vi "Decode.vi"(7 "Session Key":string, 8 "error in (no error)":errorcluster, 9 "Socket":string, 10 "Message In":string[](array[string]), 11 "object in":refnum<class "Message Class.lvclass">) -> (0 "error out":errorcluster, 1 "parent_header":T1={"msg_id"="", "username"="", "session"="", "date"=timestamp(0 s since 1904-01-01), "msg_type"="", "version"="5.0"}, 2 "Header":T1={"msg_id"="", "username"="", "session"="", "date"=timestamp(0 s since 1904-01-01), "msg_type"="", "version"="5.0"}, 3 "object out":refnum<class "Message Class.lvclass">, 4 "HMAC Signature":bool)   [LabVIEW 2018, in "ClientMessaging.lvlib" / "Message Class.lvclass"]
doc: "Decode a message and make a child class of the appropriate type"
uses:
  Message Class.lvclass
  protected/header_dict.ctl
  Message Class.lvclass/Message Class.ctl
  SHA256/SHA256.lvlib
  <vilib>/JDP Science/JSONtext/JSONtext.lvlib
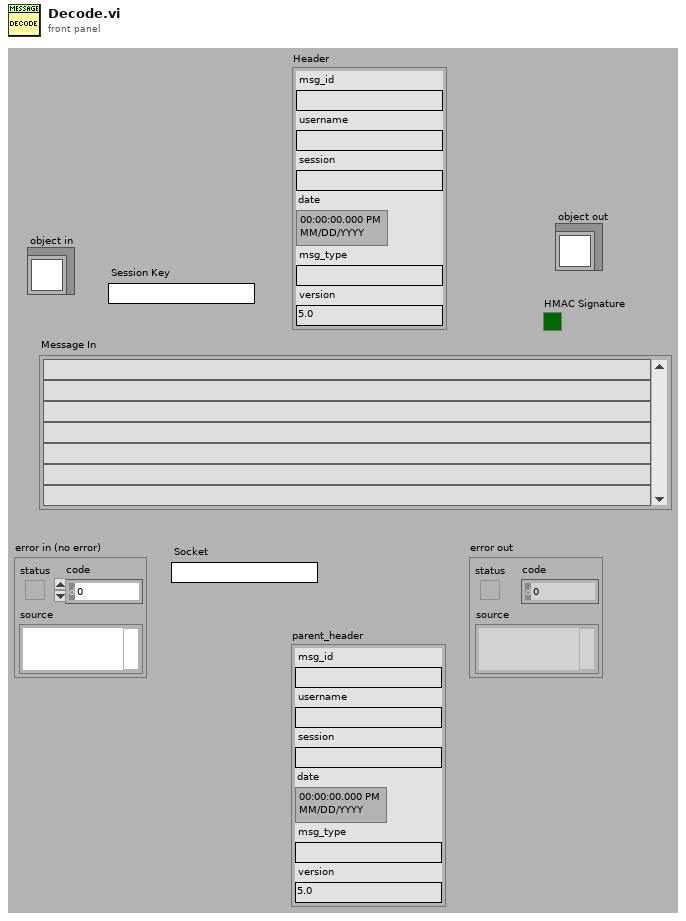
[diagram p1: front panel]
types:
  T1 = typedef "ClientMessaging.lvlib/Message Class.lvclass/header_dict.ctl" = cluster{"msg_id":string, "username":string, "session":string, "date":timestamp, "msg_type":string, "version":string}
  T2 = cluster{"[0]":string, "[1]":string, "[2]":string, "[3]":string}
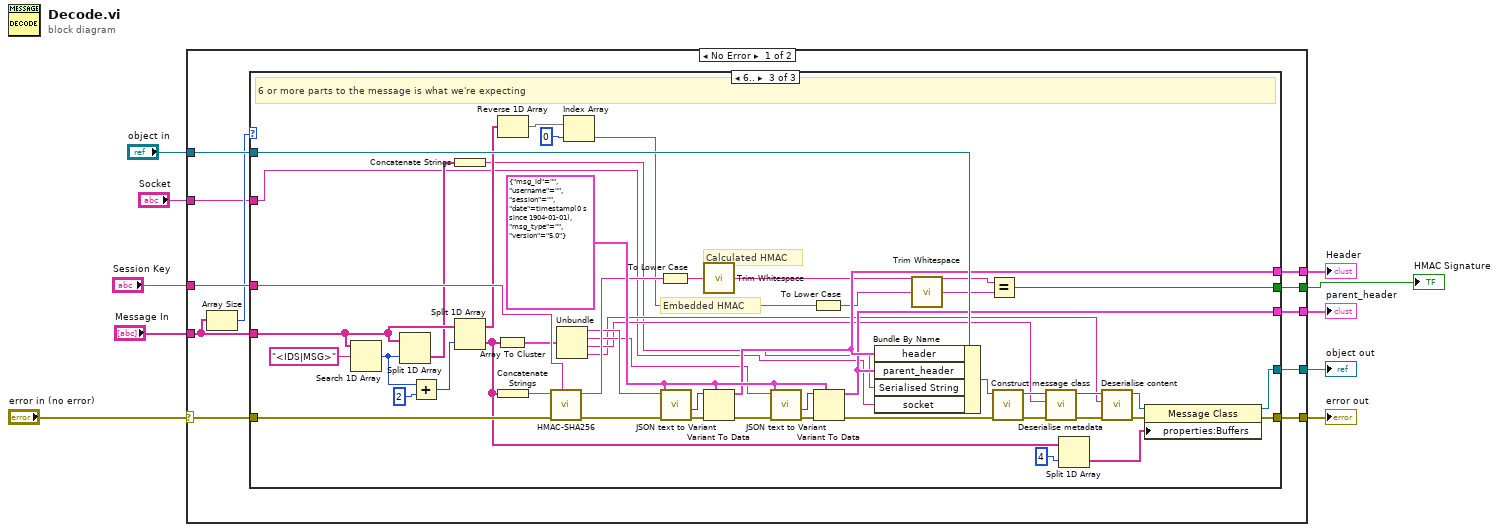
[diagram p0: block diagram]
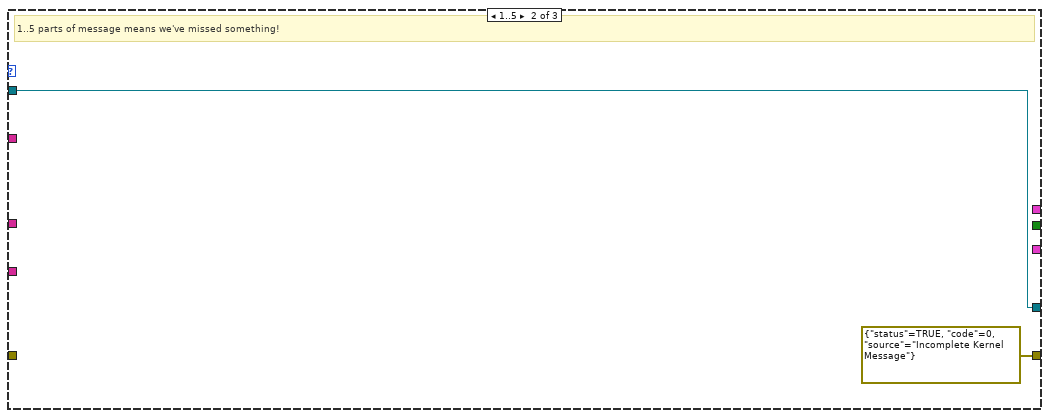
[diagram p3: hidden frame]
diagram:
  n1 = case shown="No Error" "error in (no error)" {
    selector: "error in (no error)" -> [w16 w76]
    tunnel: [w19 w76] -> w9
    tunnel: [w20 w75] -> w7
    tunnel: "object in" -> [w21 w75]
    tunnel: "Message In" -> [w13 _]
    tunnel: [w18 _] -> w5
    tunnel: [w17 _] -> w4
    tunnel: "Session Key" -> [w14 _]
    tunnel: [w15 _] -> w2
    tunnel: "Socket" -> [w11 _]
    frame No Error {
      n2 = Array Size(array=w13) -> (size(s)=w12:i32)
      n3 = case shown="6.." w12 {
        tunnel: w21 -> [w22 w25 w73]
        tunnel: [w22 w25 w59] -> w20
        tunnel: [w23 errorcluster {"status"=TRUE, "code"=0, "source"="Incomplete Kernel Message"} ("error out") w58] -> w19
        tunnel: [_ _ w57] -> w18
        tunnel: [_ _ w56] -> w17
        tunnel: w16 -> [w23 _ w55]
        tunnel: [_ _ w49] -> w15
        tunnel: w14 -> [_ _ w48]
        tunnel: w13 -> [_ _ w30]
        tunnel: w11 -> [_ _ w26]
        frame 0, Default {
          # "Ignore empty messages (probably just timeo out waiting for someone to talk to us)"
        }
        frame 1..5 {
          # "1..5 parts of message means we've missed something!"
        }
        frame 6.. {
          w66 = T1 {"msg_id"="", "username"="", "session"="", "date"=timestamp(0 s since 1904-01-01), "msg_type"="", "version"="5.0"} ("header")
          # "Calculated HMAC"
          # "Embedded HMAC"
          # "6 or more parts to the message is what we're expecting"
          n4 = Search 1D Array(1D array=w30, element="<IDS|MSG>" ("search string/char (-)")) -> (index of element=w29:i32)  [unwired: 1 in]
          n5 = Split 1D Array(array=w30, index=w29) -> (second subarray=w28:string[])  [unwired: 1 out]
          n6 = Add(x=w29, y=2) -> (x+y=w45:i32)
          n7 = Concatenate Strings(w28) -> (w27:string)
          n8 = Split 1D Array(array=w30, index=w45) -> (first subarray=w43:string[], second subarray=w33:string[])
          n9 = Array To Cluster(array=w33) -> (cluster=w39:T2)
          n10 = Reverse 1D Array(array=w43) -> (reversed array=w42:string[])
          n11 = Concatenate Strings(w33) -> (w47:string)
          n12 = call <vilib>:"HMAC-SHA256.vi"("Key"=w48, "error In"=w55, "String to Encode"=w47) -> ("error Out"=w46:errorcluster, "Hash String"=w54:string)  [unwired: 7 in]
          n13 = Unbundle(w39) -> ("[0]"=w38:string, "[1]"=w37:string, "[2]"=w36:string, "[3]"=w35:string)
          n14 = Index Array(array=w42, index=0) -> (element=w40:string)
          n15 = To Lower Case(string=w54) -> (all lower case string=w53:string)
          n16 = call <vilib>:"JSON text to Variant.vi"("error in (no error)"=w46, "Data Type"=w66, "JSON"=w38) -> ("error out"=w70:errorcluster, "Variant out"=w71:variant)  [unwired: 7 in]
          n17 = call <vilib>:"Trim Whitespace.vi"("string"=w53) -> ("trimmed string"=w51:string)  [unwired: 1 in]
          n18 = Variant To Data(error in=w70, type=w66, Variant=w71) -> (data=w57:T1, error out=w69:errorcluster)
          n19 = call <vilib>:"JSON text to Variant.vi"("error in (no error)"=w69, "Data Type"=w66, "JSON"=w37) -> ("error out"=w68:errorcluster, "Variant out"=w67:variant)  [unwired: 7 in]
          n20 = To Lower Case(string=w40) -> (all lower case string=w52:string)
          n21 = Variant To Data(error in=w68, type=w66, Variant=w67) -> (data=w56:T1, error out=w64:errorcluster)
          n22 = Bundle By Name(cluster=w73, "header"=w57, "parent_header"=w56, "Serialised String"=w27, "socket"=w26) -> (w72:refnum<class "Message Class.lvclass">)
          n23 = call <vilib>:"Trim Whitespace.vi"("string"=w52) -> ("trimmed string"=w50:string)  [unwired: 1 in]
          n24 = Equal?(x=w51, y=w50) -> (x = y?=w49:bool)
          n25 = call "Construct message class.vi"("error in (no error)"=w64, "object in"=w72) -> ("error out"=w63:errorcluster, "object out"=w65:refnum<class "Message Class.lvclass">)  [unwired: 8 in]
          n26 = call-dynamic "Deserialise metadata.vi"("error in (no error)"=w63, "JSON String to decode"=w36, "object in"=w65) -> ("error out"=w61:errorcluster, "object out"=w62:refnum<class "Message Class.lvclass">)  [unwired: 7 in]
          n27 = Split 1D Array(array=w33, index=4) -> (second subarray=w31:string[])  [unwired: 1 out]
          n28 = call-dynamic "Deserialise content.vi"("error in (no error)"=w61, "JSON String to decode"=w35, "object in"=w62) -> ("error out"=w60:errorcluster, "object out"=w34:refnum<class "Message Class.lvclass">)  [unwired: 7 in]
          n29 = property class="Message Class"(reference=w34, error in=w60, "properties:Buffers"=w31) -> (reference out=w59:refnum<class "Message Class.lvclass">, error out=w58:errorcluster)
        }
      }
    }
    frame Error {
    }
  }
  "error out" <- w9
  "object out" <- w7
  "Header" <- w5
  "parent_header" <- w4
  "HMAC Signature" <- w2
